vi "ISEG_HVChannel.constructor.vi"(0 "name":string, 2 "data in":string, 5 "error in (no error)":errorcluster) -> (14 "i ref out":refnum<vi>, 16 "data out":string, 19 "error out":errorcluster)   [LabVIEW 2014, in "ISEG_HVChannel.lvlib"]
doc: "This is the constructor of a class.\n\nLicense Agreement for this software:\n\nCopyright (C)\nGesellschaft für Schwerionenforschung, GSI\nPlanckstr. 1\n64291 Darmstadt\nGermany\n\nContact: D.Beck@gsi.de \n\nThis program is free software; you can redistribute it and/or modify it under the terms of the \nGNU General Public License as published by the Free Software Foundation; either version 2 of \nthe license, or (at your option) any later version.\n\nThis program is distributed in the hope that it will be useful, but WITHOUT ANY WARRANTY; \nwithout even the implied warranty of MERCHANTABILITY or FITNESS FOR A PARTICULAR PURPOSE. See the GNU General License for more details (http://www.gnu.org).\n\nGesellschaft für Schwerionenforschung, GSI\nPlanckstr. 1, 64291 Darmstadt, Germany\nFor all questions and ideas contact: M.Richter@gsi.de, H.Brand@gsi.de or D.Beck@gsi.de.\nLast update: 16-JUN-2004"
uses:
  ISEG_HVChannel.lvlib
  ISEG_HVChannel.i attribute.ctl
  ISEG_HVChannel.DIM Status.ctl
  CSCore/CSApplicationBaseClasses/DeviceBase/DeviceBase.myEventNames.ctl
  CSCore/CSSystem/CSSystemLib/CSSystemLib.lvlib
  CSCore/CSApplicationBaseClasses/PSChannelBase/PSChannelBase.lvlib
  CSCore/CSApplicationBaseClasses/DeviceBase/DeviceBase.lvlib
  CSCore/BaseProcess/BaseProcess.lvlib
panel:
  in  "Cluster":T1 {"Channel Array"."EventMask"."EventMask" format="%.0b"; "Channel Array"."Status"."Status" format="%.0b"}
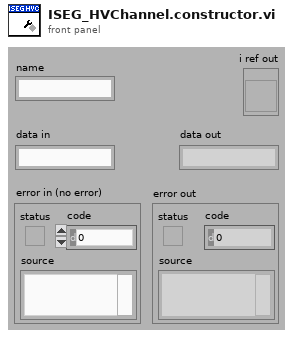
[diagram p1: front panel]
types:
  T1 = typedef "ISEG_HVChannel.lvlib/ISEG_HVChannel.i attribute.ctl" = cluster{"Channel Array":cluster{"Logical Name":string, "Address":string, "error in (no error)":errorcluster, "Status":cluster{"Status":i16, "DIM Status":T2}, "On":cluster{"On":bool, "DIM Status":T2}, "VMeas ":cluster{"VMeas":dbl, "DIM Status":T2}, "VSet ":cluster{"VSet":dbl, "DIM Status":T2}, "ITrip ":cluster{"ITrip":dbl, "DIM Status":T2}, "IMeas":cluster{"IMeas":dbl, "DIM Status":T2}, " RampSpeed":cluster{"RampSpeed":dbl, "DIM Status":T2}, "EventMask ":cluster{"EventMask":i16, "DIM Status":T2}}[], "VoltageInRangeBand":dbl, "NofCh":cluster{"NofCh":i32, "DIM Service":i32}, "BoardPrefix":string}
  T2 = typedef "ISEG_HVChannel.lvlib/ISEG_HVChannel.DIM Status.ctl" = cluster{"no link":bool, "quality":i32, "Time Stamp":timestamp}
  T3 = enum16{"SetAttribute", "GetAttribute", "CreateAttribute", "DestroyAttribute", "DestroyAllAtributes"}
  T4 = typedef "DeviceBase.lvlib/DeviceBase.myEventNames.ctl" = enum16{"lvmsg://Initialize", "lvmsg://Close", "lvmsg://Configure", "lvmsg://Reset", "lvmsg://IDQuery"}
  T5 = typedef "BaseProcess.lvlib/BaseProcess.i attribute.ctl" = cluster{"EventStatus":string, "EventError":i32, "PresetEvtWatchD":i32, "PresetPdcWatchD":i32, "EventTimeout":i32, "PeriodicInterval":i32, "Interface":string[], "Address":string[], "Special":string[], "PeriodicError":i32, "PeriodicStatus":string, "SuperProc":string, "Descriptors":T6[], "CaseRef":refnum<vi>, "PdcRef":refnum<vi>, "Thread Ref":refnum<vi>, "eventErrorID":i32, "eventStatusID":i32, "periodicErrorID":i32, "periodicStatusID":i32, "pdcCtrID":i32}
  T6 = typedef "BaseProcess.lvlib/BaseProcess.descriptor definition.ctl" = cluster{"selector":string, "descriptor":T7}
  T7 = typedef "BaseProcess.lvlib/BaseProcess.descriptor string definition.ctl" = string
  T8 = cluster{"Logical Name":string, "Address":string, "error in (no error)":errorcluster, "Status":cluster{"Status":i16, "DIM Status":T2}, "On":cluster{"On":bool, "DIM Status":T2}, "VMeas ":cluster{"VMeas":dbl, "DIM Status":T2}, "VSet ":cluster{"VSet":dbl, "DIM Status":T2}, "ITrip ":cluster{"ITrip":dbl, "DIM Status":T2}, "IMeas":cluster{"IMeas":dbl, "DIM Status":T2}, " RampSpeed":cluster{"RampSpeed":dbl, "DIM Status":T2}, "EventMask ":cluster{"EventMask":i16, "DIM Status":T2}}[]
  T9 = cluster{"Logical Name":string, "Address":string, "error in (no error)":errorcluster, "Status":cluster{"Status":i16, "DIM Status":T2}, "On":cluster{"On":bool, "DIM Status":T2}, "VMeas ":cluster{"VMeas":dbl, "DIM Status":T2}, "VSet ":cluster{"VSet":dbl, "DIM Status":T2}, "ITrip ":cluster{"ITrip":dbl, "DIM Status":T2}, "IMeas":cluster{"IMeas":dbl, "DIM Status":T2}, " RampSpeed":cluster{"RampSpeed":dbl, "DIM Status":T2}, "EventMask ":cluster{"EventMask":i16, "DIM Status":T2}}
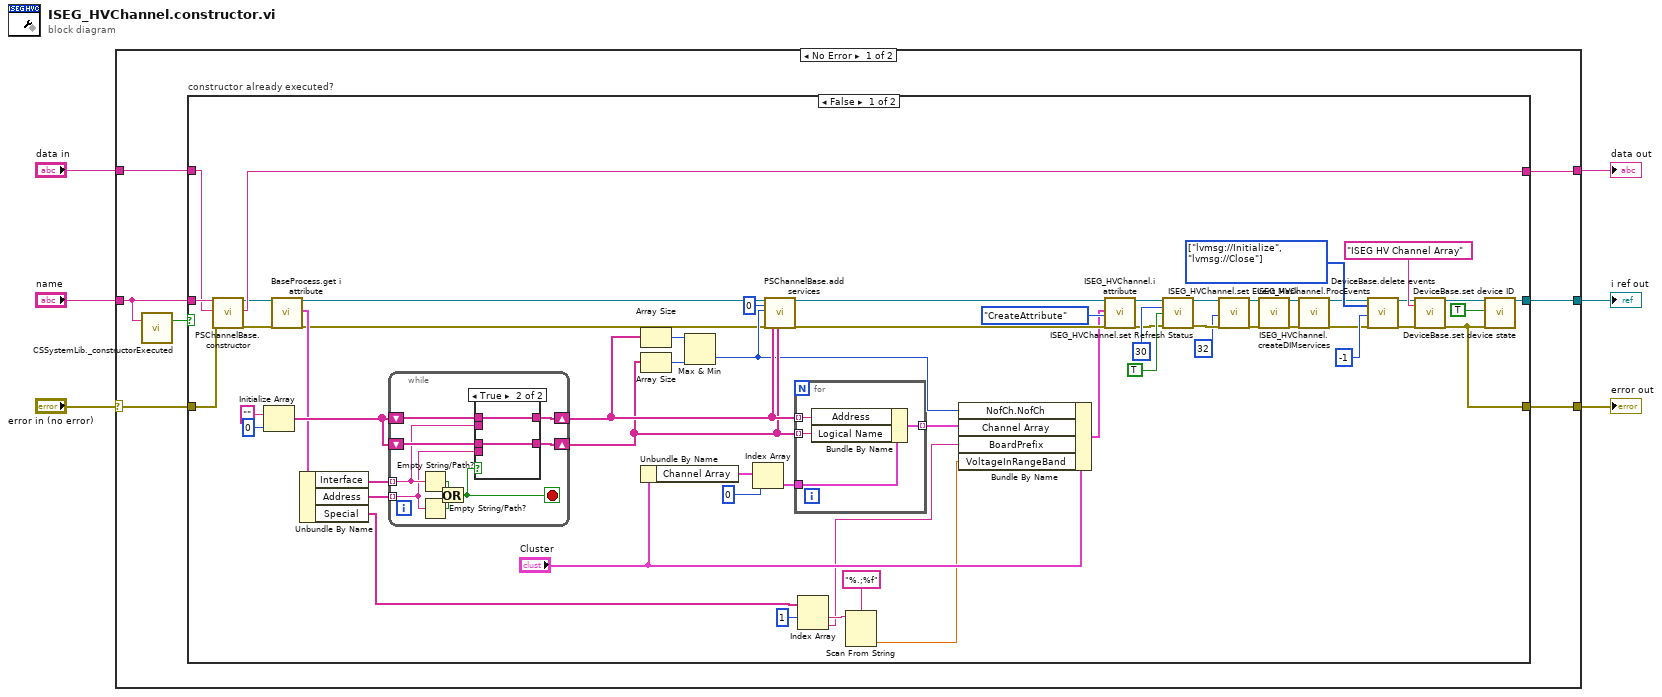
[diagram p0: block diagram]
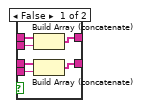
[diagram p2: hidden frame]
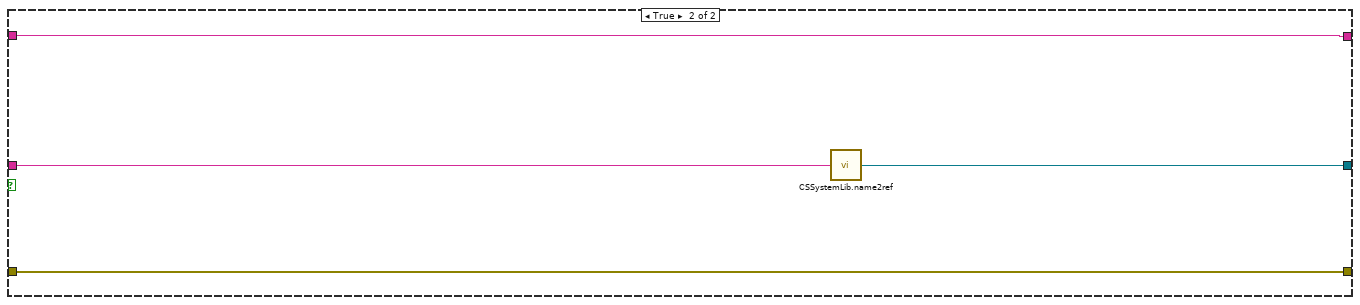
[diagram p3: hidden frame]
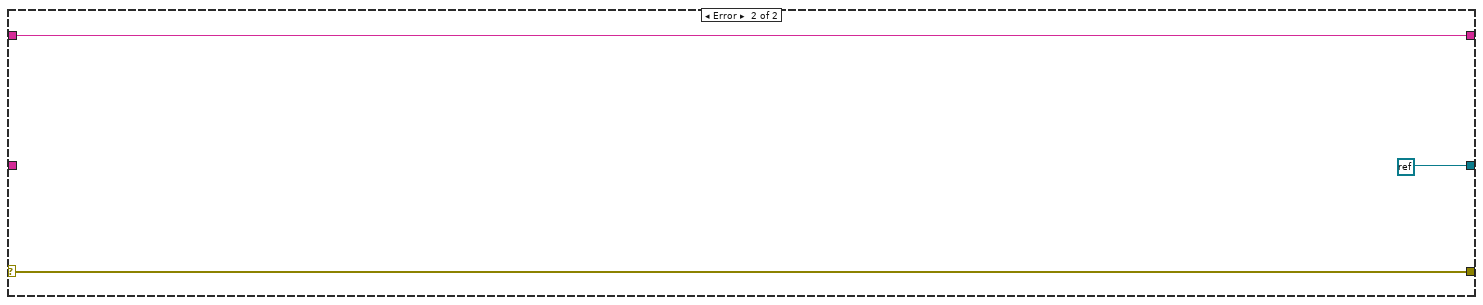
[diagram p4: hidden frame]
diagram:
  n1 = case shown="No Error" "error in (no error)" {
    selector: "error in (no error)" -> [w11 w97]
    tunnel: "name" -> [w10 _]
    tunnel: [w13 refnum<k0> refnum ("Not a Refnum Constant")] -> w5
    tunnel: [w12 w97] -> w4
    tunnel: "data in" -> [w8 w96]
    tunnel: [w7 w96] -> w1
    frame No Error {
      n2 = call "CSSystemLib._constructorExecuted.vi"("name"=w10) -> ("constructor executed?"=w9:bool)  [unwired: 18 in]
      n3 = case "constructor already executed?" shown="False" w9 {
        tunnel: w10 -> [w69 w95]
        tunnel: [w40 w94] -> w13
        tunnel: [w39 w93] -> w12
        tunnel: w11 -> [w68 w93]
        tunnel: w8 -> [w67 w92]
        tunnel: [w64 w92] -> w7
        frame False {
          w66 = T4[] [enum."lvmsg://Initialize", enum."lvmsg://Close"] items=["lvmsg://Initialize", "lvmsg://Close", "lvmsg://Configure", "lvmsg://Reset", "lvmsg://IDQuery"] ("events")
          n4 = call "PSChannelBase.constructor.vi"("name"=w69, "data in"=w67, "error in (no error)"=w68) -> ("i ref out"=w62:refnum<vi>, "data out"=w64:string, "error out"=w63:errorcluster)  [unwired: 14 in]
          n5 = Initialize Array("", 0 ("dimension size")) -> (w59:string[])
          n6 = call "BaseProcess.get i attribute.vi"("i ref in"=w62, "error in (no error)"=w63) -> ("i ref out"=w52:refnum<vi>, "i attribute"=w58:T5, "error out"=w14:errorcluster)  [unwired: 15 in]
          n7 = Unbundle By Name(w58) -> ("Interface"=w57:string[], "Address"=w56:string[], "Special"=w34:string[])
          n8 = while {
            shift-right: [w80] -> w49
            shift-left: w59 -> [w81]
            shift-right: [w78] -> w48
            shift-left: w59 -> [w79]
            tunnel: w57 -> [w77] mode=indexing
            tunnel: w56 -> [w76] mode=indexing
            stop <- w75 stop-if-true
            n9 = Empty String/Path?(string/path=w77) -> (empty?=w83:bool)
            n10 = Empty String/Path?(string/path=w76) -> (empty?=w82:bool)
            n11 = Or(x=w83, y=w82) -> (x .or. y?=w75:bool)
            n12 = case shown="True" w75 {
              tunnel: w81 -> [w89 w91]
              tunnel: [w88 w91] -> w80
              tunnel: w79 -> [w87 w90]
              tunnel: [w86 w90] -> w78
              tunnel: w77 -> [w85 _]
              tunnel: w76 -> [w84 _]
              frame False {
                n13 = Build Array (concatenate)(w89, w85) -> (w88:string[])
                n14 = Build Array (concatenate)(w87, w84) -> (w86:string[])
              }
              frame True {
              }
            }
          }
          n15 = Array Size(array=w49) -> (size(s)=w54:i32)
          n16 = Array Size(array=w48) -> (size(s)=w55:i32)
          n17 = Unbundle By Name("Cluster") -> ("Channel Array"=w44:T8)
          n18 = Max & Min(x=w54, y=w55) -> (min(x,y)=w32:i32)  [unwired: 1 out]
          n19 = Index Array(array=w44, index=0) -> (element=w43:T9)
          n20 = call "PSChannelBase.add services.vi"("i ref in"=w52, "defaultChannelIndex"=0, "nofChannels"=w32, "error in (no error)"=w14, "physicalNames"=w49, "logicalNames"=w48) -> ("i ref out"=w51:refnum<vi>, "error out"=w50:errorcluster)  [unwired: 11 in, 1 out]
          n21 = for {
            tunnel: w43 -> [w74]
            tunnel: w49 -> [w73] mode=indexing
            tunnel: w48 -> [w72] mode=indexing
            tunnel: [w71] -> w47 mode=indexing
            n22 = Bundle By Name(cluster=w74, "Address"=w73, "Logical Name"=w72) -> (w71:T9)
          }
          n23 = Index Array(array=w34, index #1=1 ("index")) -> (element #1=w33:string, element #2=w28:string)  [unwired: 1 in]
          n24 = Scan From String(format string="%.;%f", input string=w33) -> (output 1=w29:dbl)  [unwired: 3 in, 3 out]
          n25 = Bundle By Name(cluster="Cluster", "NofCh.NofCh"=w32, "Channel Array"=w47, "BoardPrefix"=w28, "VoltageInRangeBand"=w29) -> (w46:T1)
          n26 = call "ISEG_HVChannel.i attribute.vi"("VI Refnum"=w51, "CLASS.i attribute"=w46, "Action"=T3."CreateAttribute", "error in (no error)"=w50) -> ("VI Refnum out"=w19:refnum<vi>, "error out"=w20:errorcluster)  [unwired: 13 in, 1 out]
          n27 = call "ISEG_HVChannel.set Refresh Status.vi"("i ref in"=w19, "Refresh rate"=30 ("Refresh Status"), "Force"=TRUE, "error in (no error)"=w20) -> ("i ref out"=w25:refnum<vi>, "error out"=w23:errorcluster)  [unwired: 10 in]
          n28 = call "ISEG_HVChannel.set Event Mask.vi"("i ref in"=w25, "Set EventMask"=32, "error in (no error)"=w23) -> ("i ref out"=w24:refnum<vi>, "error out"=w22:errorcluster)  [unwired: 15 in]
          n29 = call "ISEG_HVChannel.ProcEvents.vi"("i ref in"=w24, "error in (no error)"=w22) -> ("i ref out"=w31:refnum<vi>, "error out"=w30:errorcluster)  [unwired: 16 in]
          n30 = call "ISEG_HVChannel.createDIMservices.vi"("i ref in"=w31, "error in"=w30) -> ("i ref out"=w18:refnum<vi>, "error out"=w16:errorcluster)  [unwired: 16 in]
          n31 = call "DeviceBase.delete events.vi"("i ref in"=w18, "events"=w66, "ms timeout (10000)"=-1, "error in (no error)"=w16) -> ("i ref out"=w17:refnum<vi>, "error out"=w15:errorcluster)  [unwired: 13 in, 1 out]
          n32 = call "DeviceBase.set device ID.vi"("i ref in"=w17, "deviceID"="ISEG HV Channel Array", "error in (no error)"=w15) -> ("i ref out"=w38:refnum<vi>, "error out"=w39:errorcluster)  [unwired: 14 in, 1 out]
          n33 = call "DeviceBase.set device state.vi"("i ref in"=w38, "implicit"=TRUE, "error in (no error)"=w39) -> ("i ref out"=w40:refnum<vi>)  [unwired: 14 in, 2 out]
        }
        frame True {
          n34 = call "CSSystemLib.name2ref.vi"("name"=w95) -> ("obj refnum"=w94:refnum<vi>)
        }
      }
    }
    frame Error {
    }
  }
  "i ref out" <- w5
  "error out" <- w4
  "data out" <- w1
